vi "Pointer producer consumer Compare Inputs.vi"(7 "ADC in":dbl[](array[numeric])=[0.0, 0.0, 0.0, 0.0], 10 "Loops":i32=1, 11 "Tolerance IN":i8) -> (0 "motor":i32, 1 "Horizontal summary":dbl, 2 "Vertical summary":dbl, 3 "Tolerance (V)":dbl)   [LabVIEW 2014]
doc: "Compare 4 inputs and display results as follows:\n\nIN0 > IN2 => MOVE DOWN [numeric \"2\"]\nIN0 < IN2 => MOVE UP [numeric \"1\"]\nIN0 = IN2 => STAY ON [numeric \"0\"] - this point also stay in position \"0\" if input values are in toleration limit\n\nIN1 > IN3 => MOVE LEFT [numeric \"1\"]\nIN1 < IN3 => MOVE RIGHT [numeric \"2\"]\nIN1 = IN3 => STAY ON [numeric \"0\"] - this point also stay in position \"0\" if input values are in toleration limit"
panel:
  out "A+":bool
  out "A-":bool caption="A+"
  out "D+":bool caption="A+"
  out "D-":bool caption="A+"
  out "U/D INDICATOR":i32
  out "L/R INDICATOR":i32
  out "A+ ADC3":dbl
  out "D+ ADC2":dbl
  out "A- ADC1":dbl
  out "D- ADC0":dbl
  # "MOTOR MOVING"
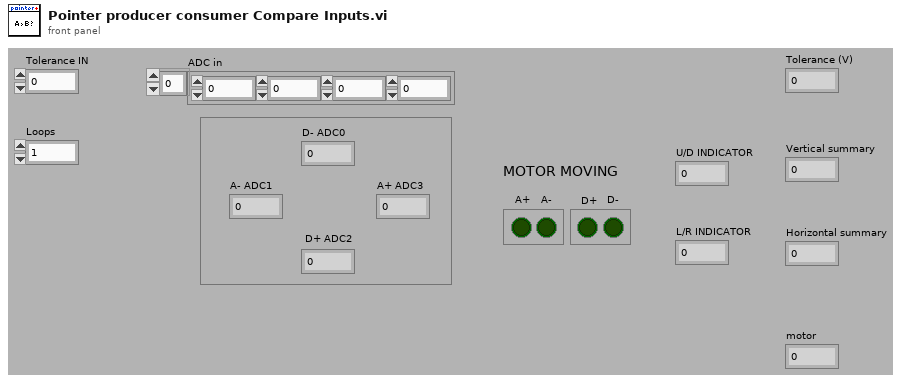
[diagram p1: front panel]
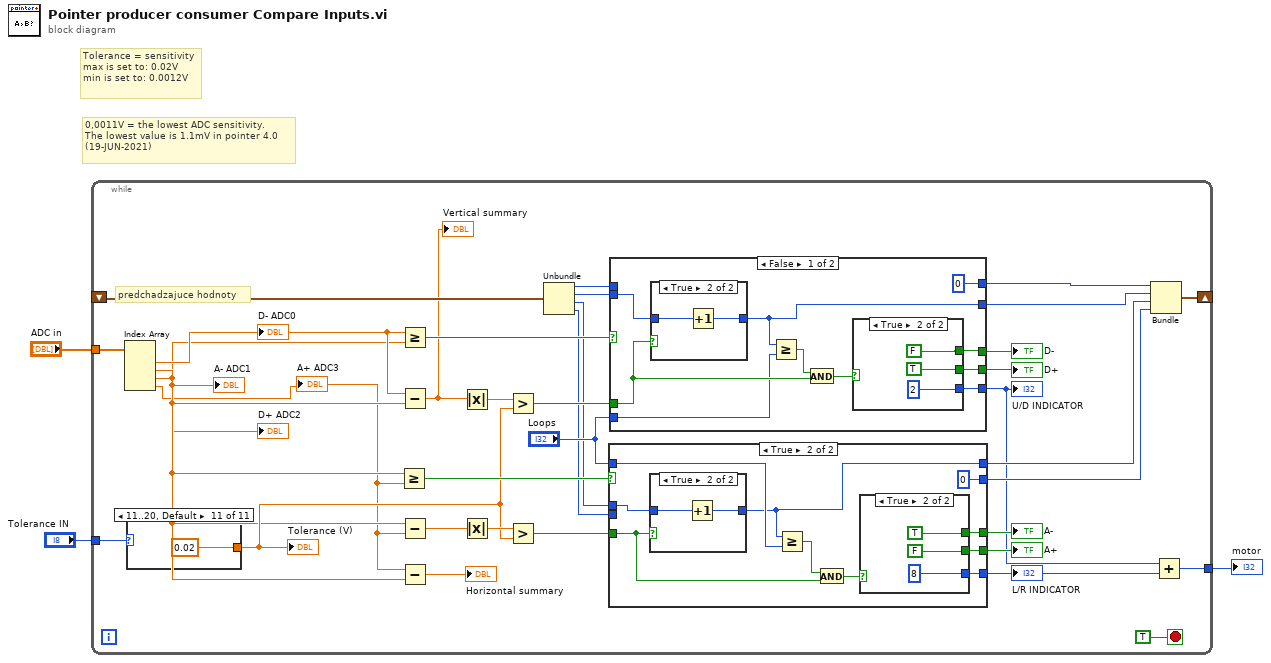
[diagram p0: block diagram]
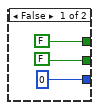
[diagram p2: hidden frame]
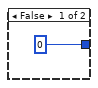
[diagram p3: hidden frame]
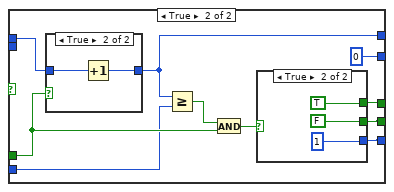
[diagram p4: hidden frame]
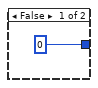
[diagram p5: hidden frame]
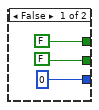
[diagram p6: hidden frame]
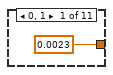
[diagram p7: hidden frame]
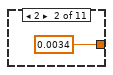
[diagram p8: hidden frame]
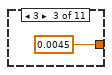
[diagram p9: hidden frame]
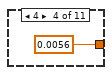
[diagram p10: hidden frame]
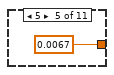
[diagram p11: hidden frame]
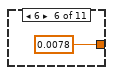
[diagram p12: hidden frame]
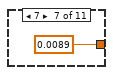
[diagram p13: hidden frame]
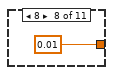
[diagram p14: hidden frame]
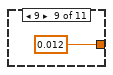
[diagram p15: hidden frame]
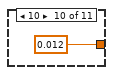
[diagram p16: hidden frame]
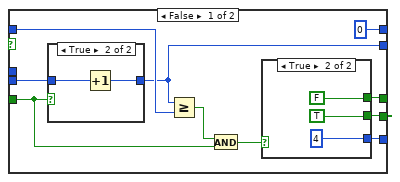
[diagram p17: hidden frame]
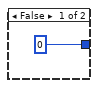
[diagram p18: hidden frame]
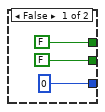
[diagram p19: hidden frame]
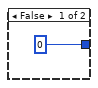
[diagram p20: hidden frame]
diagram:
  # "Tolerance = sensitivity \nmax is set to: 0.02V\nmin is set to: 0.0012V"
  # "0,0011V = the lowest ADC sensitivity. \nThe lowest value is 1.1mV in pointer 4.0 \n(19-JUN-2021)"
  n1 = while {
    tunnel: "Tolerance IN" -> [w35]
    tunnel: "ADC in" -> [w15]
    shift-right: [w22] -> _
    shift-left: _ -> [w9]
    tunnel: [w4] -> w1
    stop <- TRUE stop-if-true
    # "predchadzajuce hodnoty"
    n2 = Index Array(array=w15) -> (element #1=w14:dbl, element #2=w13:dbl, element #3=w12:dbl, element #4=w11:dbl)  [unwired: 4 in]
    "D- ADC0" <- w14
    "A- ADC1" <- w13
    "D+ ADC2" <- w12
    "A+ ADC3" <- w11
    n3 = case shown="11..20, Default" w35 {
      tunnel: [0.0023 0.0034 0.0045 0.0056 0.0067 0.0078 0.0089 0.01 0.012 0.012 0.02] -> w16
      frame 0, 1 {
      }
      frame 2 {
      }
      frame 3 {
      }
      frame 4 {
      }
      frame 5 {
      }
      frame 6 {
      }
      frame 7 {
      }
      frame 8 {
      }
      frame 9 {
      }
      frame 10 {
      }
      frame 11..20, Default {
      }
    }
    "Tolerance (V)" <- w16
    n4 = Greater Or Equal?(x=w13, y=w11) -> (x >= y?=w26:bool)
    n5 = Greater Or Equal?(x=w14, y=w12) -> (x >= y?=w31:bool)
    n6 = Subtract(x=w14, y=w12) -> (x-y=w8:dbl)
    "Vertical summary" <- w8
    n7 = Subtract(x=w13, y=w11) -> (x-y=w36:dbl)
    n8 = Subtract(x=w11, y=w13) -> (x-y=→"Horizontal summary":dbl)
    n9 = Absolute Value(x=w8) -> (abs(x)=w38:dbl)
    n10 = Absolute Value(x=w36) -> (abs(x)=w37:dbl)
    n11 = Greater?(x=w38, y=w16) -> (0:w30:bool)
    n12 = Greater?(x=w37, y=w16) -> (0:w27:bool)
    n13 = Unbundle(w9) -> (w21:i32, w20:i32, w19:i32, w18:i32)
    n14 = case shown="True" w26 {
      tunnel: [w95 w116] -> w5
      tunnel: [w97 w115] -> w34
      tunnel: [w96 w114] -> w33
      tunnel: w27 -> [w92 w111]
      tunnel: "Loops" -> [w91 w110]
      tunnel: w19 -> [_ w109]
      tunnel: w18 -> [w90 _]
      tunnel: [w89 0] -> w23
      tunnel: [0 w107] -> w24
      frame False {
        n15 = case shown="True" w92 {
          tunnel: [0 w100] -> w89
          tunnel: w90 -> [_ w99]
          frame False {
          }
          frame True {
            n16 = Increment(x=w99) -> (x+1=w100:i32)
          }
        }
        n17 = Greater Or Equal?(x=w89, y=w91) -> (x >= y?=w94:bool)
        n18 = And(x=w94, y=w92) -> (x .and. y?=w93:bool)
        n19 = case shown="True" w93 {
          tunnel: [0 4] -> w95
          tunnel: [FALSE FALSE] -> w97
          tunnel: [FALSE TRUE] -> w96
          frame False {
          }
          frame True {
          }
        }
      }
      frame True {
        n20 = case shown="True" w111 {
          tunnel: [0 w119] -> w107
          tunnel: w109 -> [_ w118]
          frame False {
          }
          frame True {
            n21 = Increment(x=w118) -> (x+1=w119:i32)
          }
        }
        n22 = Greater Or Equal?(x=w107, y=w110) -> (x >= y?=w113:bool)
        n23 = And(x=w113, y=w111) -> (x .and. y?=w112:bool)
        n24 = case shown="True" w112 {
          tunnel: [0 8] -> w116
          tunnel: [FALSE TRUE] -> w115
          tunnel: [FALSE FALSE] -> w114
          frame False {
          }
          frame True {
          }
        }
      }
    }
    "L/R INDICATOR" <- w5
    "A-" <- w34
    "A+" <- w33
    n25 = case shown="False" w31 {
      tunnel: [w46 w65] -> w32
      tunnel: [w45 w64] -> w6
      tunnel: w30 -> [w43 w62]
      tunnel: [w44 w63] -> w29
      tunnel: "Loops" -> [w42 w61]
      tunnel: w20 -> [w41 _]
      tunnel: [0 w60] -> w25
      tunnel: [w39 0] -> w17
      tunnel: w21 -> [_ w58]
      frame False {
        n26 = case shown="True" w43 {
          tunnel: [0 w57] -> w39
          tunnel: w41 -> [_ w56]
          frame False {
          }
          frame True {
            n27 = Increment(x=w56) -> (x+1=w57:i32)
          }
        }
        n28 = Greater Or Equal?(x=w39, y=w42) -> (x >= y?=w48:bool)
        n29 = And(x=w48, y=w43) -> (x .and. y?=w47:bool)
        n30 = case shown="True" w47 {
          tunnel: [0 ("Numeric") 2] -> w45
          tunnel: [FALSE TRUE] -> w46
          tunnel: [FALSE FALSE] -> w44
          frame False {
          }
          frame True {
          }
        }
      }
      frame True {
        n31 = case shown="True" w62 {
          tunnel: [0 w70] -> w60
          tunnel: w58 -> [_ w69]
          frame False {
          }
          frame True {
            n32 = Increment(x=w69) -> (x+1=w70:i32)
          }
        }
        n33 = Greater Or Equal?(x=w60, y=w61) -> (x >= y?=w66:bool)
        n34 = And(x=w66, y=w62) -> (x .and. y?=w67:bool)
        n35 = case shown="True" w67 {
          tunnel: [0 ("Numeric") 1] -> w64
          tunnel: [FALSE FALSE] -> w65
          tunnel: [FALSE TRUE] -> w63
          frame False {
          }
          frame True {
          }
        }
      }
    }
    "U/D INDICATOR" <- w6
    "D-" <- w29
    "D+" <- w32
    n36 = Bundle(w25, w17, w24, w23) -> (w22:cluster{i32, i32, i32, i32})  [unwired: 1 in]
    n37 = Add(x=w6, y=w5) -> (x+y=w4:i32)
  }
  "motor" <- w1
